vi "Get Single.vi"(0 "Session Handle in":T1, 5 "CMD":string="R1", 11 "error in":errorcluster) -> (4 "Session Handle out":T1, 6 "DataOut":sgl, 15 "error out":errorcluster)   [LabVIEW 2018, in "Serial Session.lvclass"]
doc: "Write to serial port and retrieve a floating point number."
uses:
  Serial Session.lvclass
  Typedefs/Session Handle.ctl
  Asynchronous Write.vi
  Asynchronous Read.vi
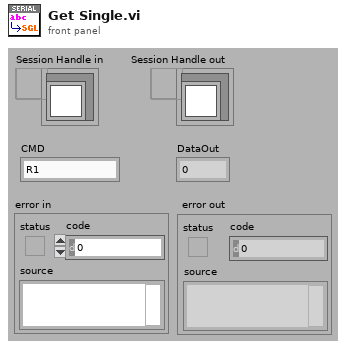
[diagram p1: front panel]
types:
  T1 = typedef "Serial Session.lvclass/Session Handle.ctl" = refnum<data-value>
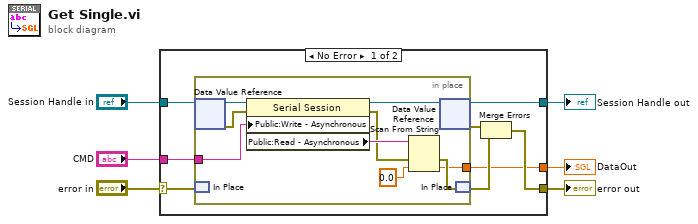
[diagram p0: block diagram]
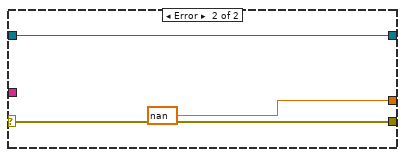
[diagram p2: hidden frame]
diagram:
  n1 = case shown="No Error" "error in" {
    selector: "error in" -> [w9 w25]
    tunnel: "Session Handle in" -> [w14 w26]
    tunnel: [w13 w26] -> w5
    tunnel: [w10 w25] -> w4
    tunnel: "CMD" -> [w8 _]
    tunnel: [w7 sgl nan ("default value 1")] -> w1
    frame No Error {
      n2 = in-place {
        in-place-border: w8 -> [w17]
        in-place-border: [w15] -> w7
        n3 = in-place-dvr #1(w14) -> (w19:refnum<class "Serial Session.lvclass">, w20:errorcluster)
        n4 = in-place-match #2(w9) -> ()  [unwired: 1 out]
        n5 = property class="Serial Session"(reference=w19, error in=w20, "Public:Write - Asynchronous"=w17) -> (reference out=w18:refnum<class "Serial Session.lvclass">, error out=w22:errorcluster, "Public:Read - Asynchronous"=w23:string)
        n6 = Scan From String(input string=w23, error in=w22, default 1=sgl 0.0 ("default value 1")) -> (error out=w16:errorcluster, output 1=w15:sgl)  [unwired: 2 in, 2 out]
        n7 = in-place-dvr #1(w18) -> (w13:T1, w11:errorcluster)
        n8 = in-place-match #2(w16) -> (w12:errorcluster)
      }
      n9 = Merge Errors(w11, w12) -> (w10:errorcluster)
    }
    frame Error {
    }
  }
  "Session Handle out" <- w5
  "error out" <- w4
  "DataOut" <- w1
